vi "PicoScope2000Close.vi"(4 "error in":errorcluster, 7 "handle":i16=1) -> (0 "error out":errorcluster, 3 "handle out":i16)   [LabVIEW 2010]
doc: "This closes the oscilloscope and should be called before exiting an application."
uses:
  ps2000.dll
panel:
  out "return":i16
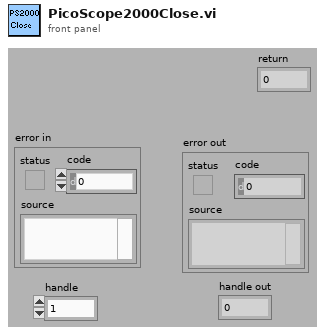
[diagram p1: front panel]
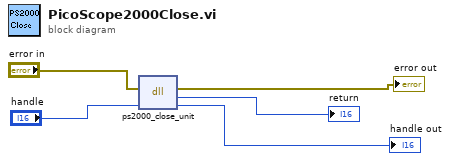
[diagram p0: block diagram]
diagram:
  n1 = dll-call lib="ps2000.dll" fn="ps2000_close_unit" ("ps3000.dll:_ps3000_open_unit@0")(error in="error in", "handle"="handle") -> (error out=→"error out":errorcluster, "return"=→"return":i16, "handle"=→"handle out":i16)  [unwired: 2 in, 1 out]
